vi "Read Data Bus.vi"(8 "error in (no error)":errorcluster, 11 "IO in":refnum<class "IO.lvclass">) -> (0 "error out":errorcluster, 3 "Data":u8 format="%02x")   [LabVIEW 2021, in "IO.lvclass"]
uses:
  IO.lvclass
  IO.lvclass/IO.ctl
  <vilib>/DAQmx/read.llb/DAQmx Read (Digital 1D Bool NChan 1Samp 1Line).vi
  <vilib>/DAQmx/miscellaneous.llb/DAQmx Fill In Error Info.vi
  <resource>/objmgr/daqmx.rc
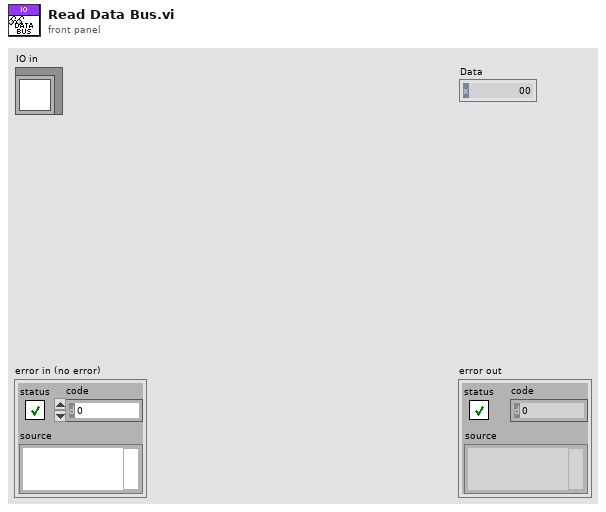
[diagram p1: front panel]
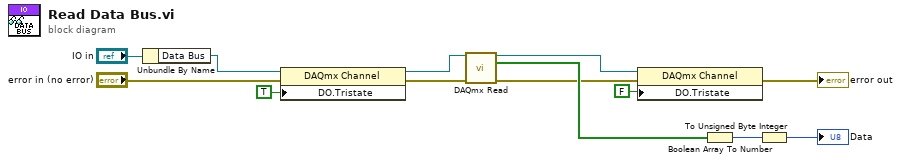
[diagram p0: block diagram]
diagram:
  n1 = Unbundle By Name("IO in") -> ("Data Bus"=w3:refnum<k21>)
  n2 = property class="DAQmx Channel"(reference=w3, error in="error in (no error)", "DO.Tristate"=TRUE) -> (reference out=w12:refnum<k21>, error out=w5:errorcluster)
  n3 = call-poly <vilib>:"DAQmx Read.vi"("task/channels in"=w12, "error in"=w5) -> ("task out"=w11:refnum<k21>, "data"=w8:bool[], "error out"=w4:errorcluster)  [unwired: 11 in]
  n4 = property class="DAQmx Channel"(reference=w11, error in=w4, "DO.Tristate"=FALSE) -> (error out=→"error out":errorcluster)  [unwired: 1 out]
  n5 = Boolean Array To Number(Boolean array=w8) -> (number=w2:u32)
  n6 = To Unsigned Byte Integer(number=w2) -> (unsigned 8bit integer=→"Data":u8)
